vi "Serial.vi"() -> ()   [LabVIEW 2020]
uses:
  <vilib>/Instr/_visa.llb/VISA Configure Serial Port (Instr).vi
panel:
  out "read buffer":string
  out "error out":errorcluster
  in  "stop":bool
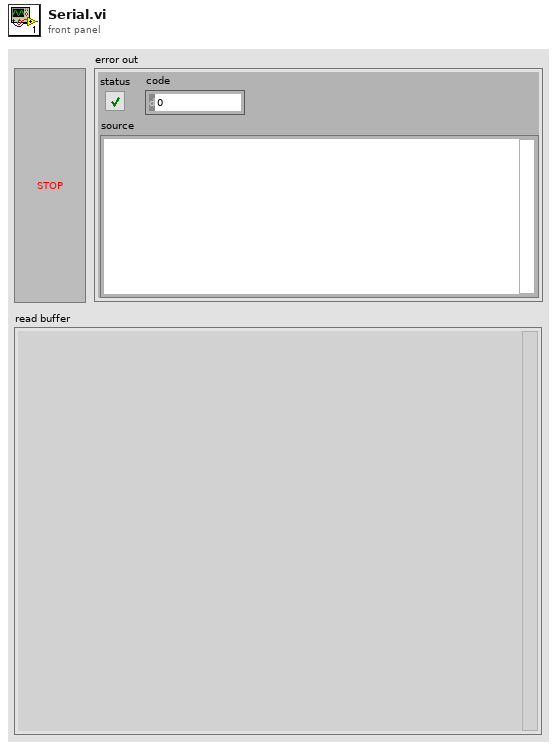
[diagram p1: front panel]
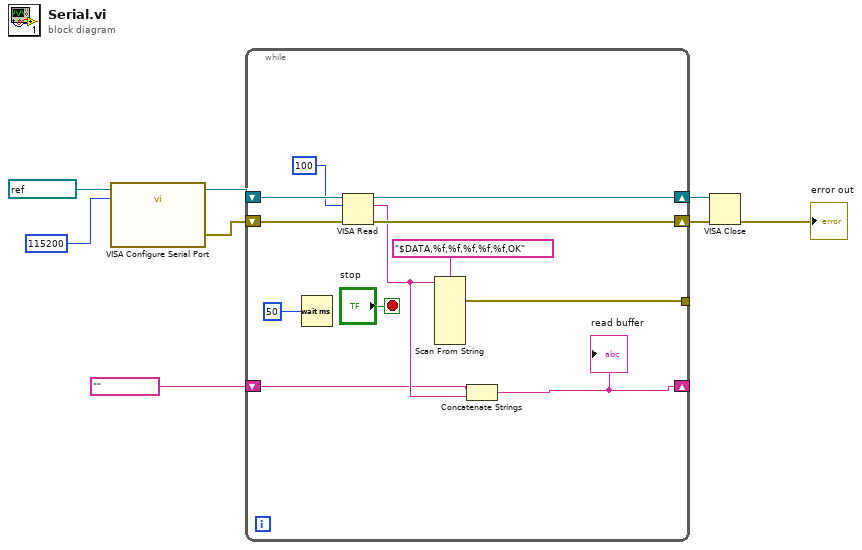
[diagram p0: block diagram]
diagram:
  n1 = call-poly "VISA Configure Serial Port"("VISA resource name"=refnum<visa-resource-name> "COM15", "baud rate (9600)"=u32 115200) -> ("VISA resource name out"=w8:refnum<visa-resource-name>, "error out"=w7:errorcluster)  [unwired: 12 in]
  n2 = while {
    shift-right: [w18] -> w5
    shift-left: w8 -> [w20]
    shift-right: [w13] -> w6
    shift-left: w7 -> [w19]
    tunnel: [w12] -> _
    shift-right: [w9] -> _
    shift-left: "" -> [w10]
    stop <- "stop" stop-if-true
    n3 = Wait (ms)(milliseconds to wait=u32 50) -> ()  [unwired: 1 out]
    n4 = VISA Read(VISA resource name=w20, byte count=u32 100, error in (no error)=w19) -> (VISA resource name out=w18:refnum<visa-resource-name>, read buffer=w11:string, error out=w13:errorcluster)  [unwired: 1 out]
    n5 = Scan From String(format string="$DATA,%f,%f,%f,%f,%f,OK", input string=w11) -> (error out=w12:errorcluster)  [unwired: 12 in, 2 out]
    n6 = Concatenate Strings(w10, w11) -> (w9:string)
    "read buffer" <- w9
  }
  n7 = VISA Close(VISA resource name=w5, error in (no error)=w6) -> (error out=→"error out":errorcluster)
